vi "Check Status (No Objects).vi"(8 "error in (no error)":errorcluster, 11 "Cluster In":T1={"Arming (Trigger) Source"=2, "Pulse Mode"=2, "Overall Period"=0.0, "Ch1Delay"=0.0, "Ch1Width"=0.0, "Ch2Delay"=0.0, "Ch2Width"=0.0, "Output Levels"={"1 High"=0.0, "1 Low"=0.0, "2 High"=0.0, "2 Low"=0.0}, "Outputs 1/!1/2/!2 "=[], "Bit Period"=0.0, "Ch1 Pattern"="", "Ch2 Pattern"="", "Strobe Pattern"="", "Ch1Width(true)"=FALSE, "Ch2Width(true)"=FALSE} {"Arming (Trigger) Source" items=["Immediate (Continuous Mode)", "Internal PLL", "External", "Manual"]; "Pulse Mode" items=["Pulses", "Pattern"]}) -> (0 "error out":errorcluster, 1 "Status":string, 2 "Ready?":bool, 3 "Cluster Out":T1={"Arming (Trigger) Source"=2, "Pulse Mode"=2, "Overall Period"=0.0, "Ch1Delay"=0.0, "Ch1Width"=0.0, "Ch2Delay"=0.0, "Ch2Width"=0.0, "Output Levels"={"1 High"=0.0, "1 Low"=0.0, "2 High"=0.0, "2 Low"=0.0}, "Outputs 1/!1/2/!2 "=[], "Bit Period"=0.0, "Ch1 Pattern"="", "Ch2 Pattern"="", "Strobe Pattern"="", "Ch1Width(true)"=FALSE, "Ch2Width(true)"=FALSE} {"Arming (Trigger) Source" items=["Immediate (Continuous Mode)", "Internal PLL", "External", "Manual"]; "Pulse Mode" items=["Pulses", "Pattern"]})   [LabVIEW 2009]
doc: "Checks if the instrument is powered on and updates its member data with the instrument's current status."
uses:
  Global/GPIB Numbers.vi
  Pulse Generator.lvclass
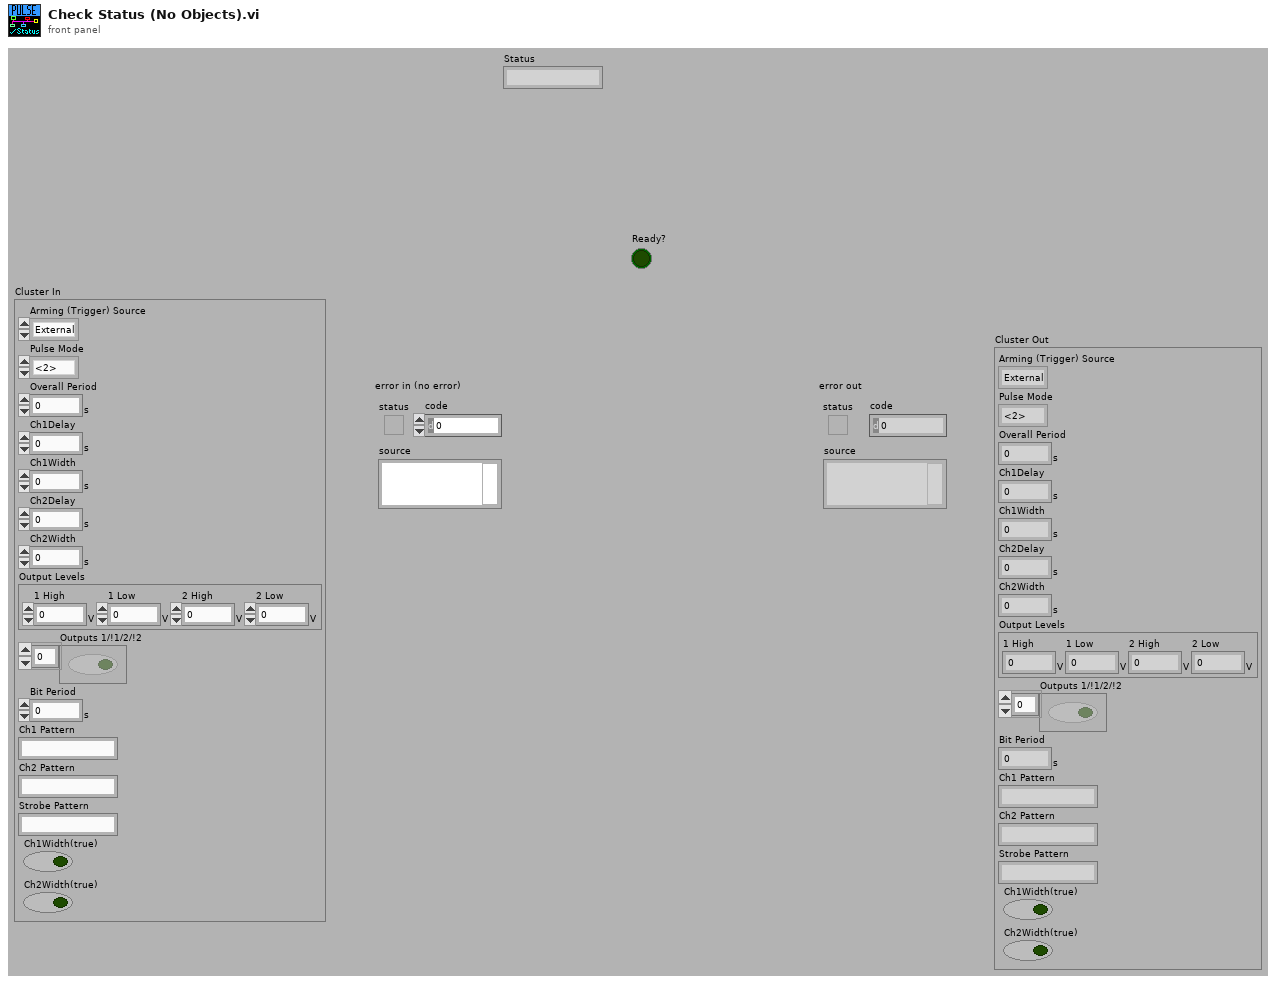
[diagram p1: front panel]
types:
  T1 = cluster{"Arming (Trigger) Source":u16, "Pulse Mode":u16, "Overall Period":dbl[unit], "Ch1Delay":dbl[unit], "Ch1Width":dbl[unit], "Ch2Delay":dbl[unit], "Ch2Width":dbl[unit], "Output Levels":cluster{"1 High":dbl[unit], "1 Low":dbl[unit], "2 High":dbl[unit], "2 Low":dbl[unit]}, "Outputs 1/!1/2/!2 ":bool[], "Bit Period":dbl[unit], "Ch1 Pattern":string, "Ch2 Pattern":string, "Strobe Pattern":string, "Ch1Width(true)":bool, "Ch2Width(true)":bool}
  T2 = enum16{"Invalid", "Channel 1", "Channel 2", "Strobe"}
  T3 = typedef "GPIB Type Def.ctl" = cluster{"Name":string, "bus":dbl, "GPIB":dbl, "GPIB as string":string, "byte":i32, "VISA Resource Name":refnum<visa-resource-name>}
  T4 = enum16{"Immediate (Continuous Mode)", "Internal PLL", "External", "Manual"}
  T5 = enum32{"Continuous Pulsed", "Continuous Pattern", "Internal Triggered Pattern", "External Triggered Pulsed", "External Triggered Pattern", "Other"}
  T6 = cluster{"Value High":dbl[unit], "Value Low":dbl[unit], "Value High":dbl[unit], "Value Low":dbl[unit]}
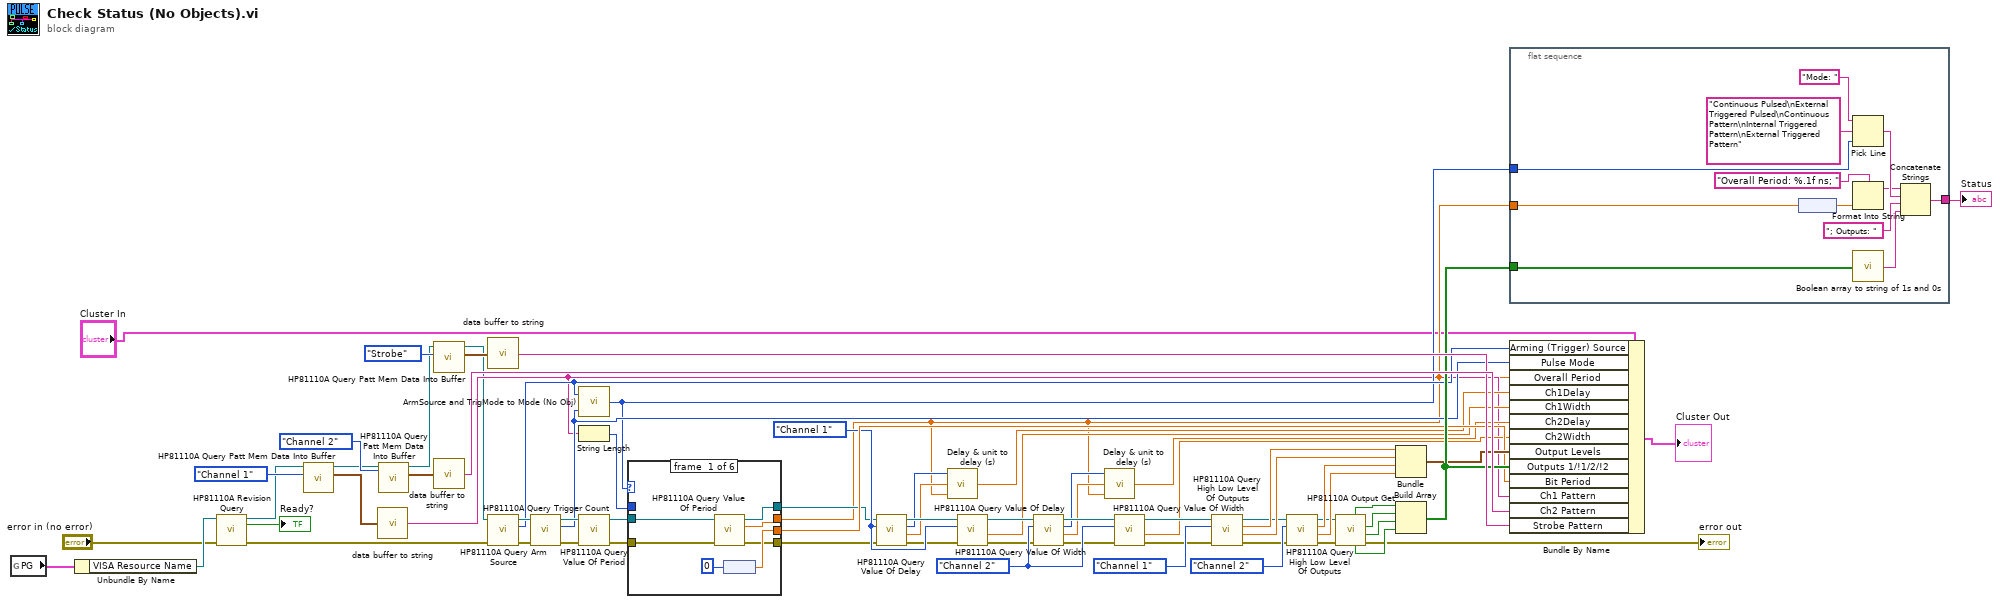
[diagram p0: block diagram]
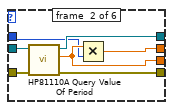
[diagram p2: hidden frame]
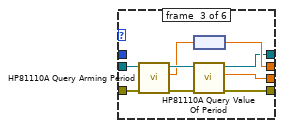
[diagram p3: hidden frame]
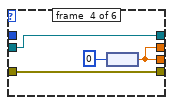
[diagram p4: hidden frame]
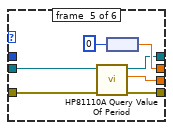
[diagram p5: hidden frame]
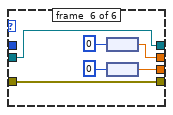
[diagram p6: hidden frame]
diagram:
  w34 = enum16{"Invalid", "Channel 1", "Channel 2"}."Channel 2" ("Channel (1:Channel 1)")
  w35 = enum16{"Invalid", "Channel 1", "Channel 2"}."Channel 1" ("Channel (1:Channel 1)")
  n1 = global read "GPIB Numbers.vi" "PG"() -> (w6:T3)
  n2 = Unbundle By Name(w6) -> ("VISA Resource Name"=w5:refnum<visa-resource-name>)
  n3 = call "HP81110A Revision Query.vi"("VISA session"=w5, "error in (no error)"="error in (no error)") -> ("dup VISA session"=w16:refnum<visa-resource-name>, "Ready?"=→"Ready?":bool, "error out"=w23:errorcluster)  [unwired: 11 out]
  n4 = call "HP81110A Query Patt Mem Data Into Buffer.vi"("Channel (1:Channel 1)"=T2."Channel 1", "VISA session"=w16) -> ("output pattern"=w54:digitaldata, "dup VISA session"=w56:refnum<visa-resource-name>)  [unwired: 1 in, 7 out]
  n5 = call "data buffer to string.vi"("output pattern"=w54) -> ("initial string"=w18:string)
  n6 = call "HP81110A Query Patt Mem Data Into Buffer.vi"("Channel (1:Channel 1)"=T2."Channel 2", "VISA session"=w56) -> ("output pattern"=w53:digitaldata, "dup VISA session"=w55:refnum<visa-resource-name>)  [unwired: 1 in, 7 out]
  n7 = call "HP81110A Query Patt Mem Data Into Buffer.vi"("Channel (1:Channel 1)"=T2."Strobe", "VISA session"=w55) -> ("output pattern"=w52:digitaldata, "dup VISA session"=w15:refnum<visa-resource-name>)  [unwired: 1 in, 7 out]
  n8 = call "data buffer to string.vi"("output pattern"=w53) -> ("initial string"=w51:string)
  n9 = call "data buffer to string.vi"("output pattern"=w52) -> ("initial string"=w50:string)
  n10 = call "HP81110A Query Arm Source.vi"("error in (no error)"=w23, "VISA session"=w15) -> ("error out"=w22:errorcluster, "Arming (Trigger) Source (0:Internal PLL)"=w40:T4, "dup VISA session"=w45:refnum<visa-resource-name>)  [unwired: 7 out]
  n11 = call "HP81110A Query Trigger Count.vi"("error in (no error)"=w22, "VISA session"=w45) -> ("error out"=w21:errorcluster, "Pulse Mode"=w39:enum16{"Pulses", "Pattern"}, "dup VISA session"=w44:refnum<visa-resource-name>)  [unwired: 7 out]
  n12 = call "ArmSource and TrigMode to Mode (No Obj).vi"("Pulse Mode"=w39, "Arming (Trigger) Source (0:Internal PLL)"=w40) -> ("Modes (changes immediately)"=w19:T5)
  n13 = String Length(string=w18) -> (length=w17:i32)
  n14 = call "HP81110A Query Value Of Period.vi"("error in (no error)"=w21, "VISA session"=w44) -> ("error out"=w20:errorcluster, "dup VISA session"=w41:refnum<visa-resource-name>)  [unwired: 1 in, 7 out]
  n15 = case shown="\"Internal Triggered Pattern\"" w19 {
    tunnel: [w76 w83 w89 w96 w102 w107] -> w14
    tunnel: [w75 w84 w90 w96 w103 w108] -> w42
    tunnel: w41 -> [w74 w82 w88 w95 w101 w106]
    tunnel: [w73 w81 w87 w94 w100 w105] -> w13
    tunnel: [w72 w80 w86 w95 w99 w106] -> w32
    tunnel: w20 -> [w71 w79 w85 w94 w98 w105]
    tunnel: w17 -> [_ w78 _ _ _ _]
    frame #0 {
      n16 = call "HP81110A Query Value Of Period.vi"("error in (no error)"=w71, "VISA session"=w74) -> ("error out"=w73:errorcluster, "Period Value"=w76:dbl[unit], "dup VISA session"=w72:refnum<visa-resource-name>)  [unwired: 7 out]
      n17 = node(0) -> (w75:dbl[unit])
    }
    frame #1 {
      n18 = call "HP81110A Query Value Of Period.vi"("error in (no error)"=w79, "VISA session"=w82) -> ("error out"=w81:errorcluster, "Period Value"=w84:dbl[unit], "dup VISA session"=w80:refnum<visa-resource-name>)  [unwired: 7 out]
      n19 = Multiply(x=w84, y=w78) -> (x*y=w83:dbl[unit])
    }
    frame #2 {
      n20 = call "HP81110A Query Arming Period.vi"("error in (no error)"=w85, "VISA session"=w88) -> ("error out"=w93:errorcluster, "Period Value (Sec)"=w91:dbl, "dup VISA session"=w92:refnum<visa-resource-name>)  [unwired: 7 out]
      n21 = node(w91) -> (w89:dbl[unit])
      n22 = call "HP81110A Query Value Of Period.vi"("error in (no error)"=w93, "VISA session"=w92) -> ("error out"=w87:errorcluster, "Period Value"=w90:dbl[unit], "dup VISA session"=w86:refnum<visa-resource-name>)  [unwired: 7 out]
    }
    frame #3 {
      n23 = node(0) -> (w96:dbl[unit])
    }
    frame #4 {
      n24 = call "HP81110A Query Value Of Period.vi"("error in (no error)"=w98, "VISA session"=w101) -> ("error out"=w100:errorcluster, "Period Value"=w103:dbl[unit], "dup VISA session"=w99:refnum<visa-resource-name>)  [unwired: 7 out]
      n25 = node(0) -> (w102:dbl[unit])
    }
    frame #5 {
      n26 = node(0) -> (w107:dbl[unit])
      n27 = node(0) -> (w108:dbl[unit])
    }
  }
  n28 = call "HP81110A Query Value Of Delay.vi"("error in (no error)"=w13, "Channel (1:Channel 1)"=w35, "VISA session"=w32) -> ("error out"=w12:errorcluster, "Delay Value"=w30:dbl, "Delay Unit"=w31:u16, "dup VISA session"=w36:refnum<visa-resource-name>)  [unwired: 5 out]
  n29 = call "Delay & unit to delay (s).vi"("OverallPeriod"=w14, "Delay Value"=w30, "Delay Unit"=w31) -> ("Delay (s)"=w29:dbl[unit])
  n30 = call "HP81110A Query Value Of Width.vi"("error in (no error)"=w12, "Channel (1:Channel 1)"=w35, "VISA session"=w36) -> ("error out"=w11:errorcluster, "Width Value (Sec)"=w28:dbl[unit], "dup VISA session"=w38:refnum<visa-resource-name>)  [unwired: 6 out]
  n31 = call "HP81110A Query Value Of Delay.vi"("error in (no error)"=w11, "Channel (1:Channel 1)"=w34, "VISA session"=w38) -> ("error out"=w10:errorcluster, "Delay Value"=w26:dbl, "Delay Unit"=w27:u16, "dup VISA session"=w37:refnum<visa-resource-name>)  [unwired: 5 out]
  n32 = call "Delay & unit to delay (s).vi"("OverallPeriod"=w14, "Delay Value"=w26, "Delay Unit"=w27) -> ("Delay (s)"=w25:dbl[unit])
  n33 = call "HP81110A Query Value Of Width.vi"("error in (no error)"=w10, "Channel (1:Channel 1)"=w34, "VISA session"=w37) -> ("error out"=w9:errorcluster, "Width Value (Sec)"=w24:dbl[unit], "dup VISA session"=w33:refnum<visa-resource-name>)  [unwired: 6 out]
  n34 = call "HP81110A Query High Low Level Of Outputs.vi"("error in (no error)"=w9, "Channel (1:Channel 1)"=enum16{"Invalid", "Channel 1", "Channel 2"}."Channel 1", "VISA session"=w33) -> ("error out"=w8:errorcluster, "Value Low"=w64:dbl[unit], "Value High"=w65:dbl[unit], "dup VISA session"=w47:refnum<visa-resource-name>)  [unwired: 1 in, 4 out]
  n35 = call "HP81110A Query High Low Level Of Outputs.vi"("error in (no error)"=w8, "Channel (1:Channel 1)"=enum16{"Invalid", "Channel 1", "Channel 2"}."Channel 2", "VISA session"=w47) -> ("error out"=w7:errorcluster, "Value Low"=w62:dbl[unit], "Value High"=w63:dbl[unit], "dup VISA session"=w46:refnum<visa-resource-name>)  [unwired: 1 in, 4 out]
  n36 = call "HP81110A Output Get.vi"("error in (no error)"=w7, "VISA session"=w46) -> ("error out"=→"error out":errorcluster, "output2OUT"=w69:bool, "notoutput1OUT"=w68:bool, "notoutput2OUT"=w70:bool, "output1OUT"=w67:bool)  [unwired: 5 out]
  n37 = Bundle("Value High"=w65, "Value Low"=w64, "Value High"=w63, "Value Low"=w62) -> (w48:T6)  [unwired: 1 out]
  n38 = Build Array(w67, w68, w69, w70) -> (w49:bool[])
  n39 = flat-sequence {
    tunnel: w49 -> [w113]
    tunnel: w14 -> [w117]
    tunnel: [w116] -> w43
    tunnel: w19 -> [w115]
    frame #0 {
      n40 = node(w117) -> (w121:dbl)
      n41 = Pick Line(string ("")="Mode: ", multi-line string="Continuous Pulsed\nExternal Triggered Pulsed\nContinuous Pattern\nInternal Triggered Pattern\nExternal Triggered Pattern", line index=w115) -> (output string=w119:string)
      n42 = Format Into String(format string="Overall Period: %.1f ns; ", w121) -> (resulting string=w118:string)  [unwired: 2 in, 1 out]
      n43 = call "Boolean array to string of 1s and 0s.vi"("Array"=w113) -> ("String"=w112:string)
      n44 = Concatenate Strings(w118, w119, "; Outputs: ", w112) -> (w116:string)
    }
  }
  n45 = Bundle By Name(cluster="Cluster In", "Arming (Trigger) Source"=w40, "Pulse Mode"=w39, "Overall Period"=w14, "Ch1Delay"=w29, "Ch1Width"=w28, "Ch2Delay"=w25, "Ch2Width"=w24, "Output Levels"=w48, "Outputs 1/!1/2/!2"=w49, "Bit Period"=w42, "Ch1 Pattern"=w18, "Ch2 Pattern"=w51, "Strobe Pattern"=w50) -> (→"Cluster Out":T1)
  "Status" <- w43
